vi "Speed_Ramp_test.vi"(3 "MaxRampRate":dbl, 4 "Input":dbl) -> (1 "Output":dbl)   [LabVIEW 2019]
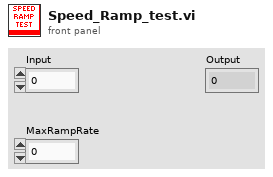
[diagram p1: front panel]
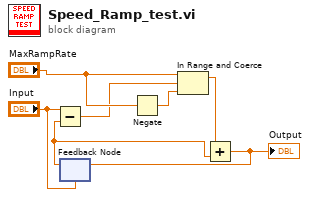
[diagram p0: block diagram]
diagram:
  n1 = feedback #1("Input") -> (w1:dbl)
  n2 = Subtract(x="Input", y=w1) -> (x-y=w5:dbl)
  n3 = Negate(x="MaxRampRate") -> (-x=w7:dbl)
  n4 = In Range and Coerce(upper limit="MaxRampRate", x=w5, lower limit=w7) -> (coerced(x)=w2:dbl)  [unwired: 1 out]
  n5 = Add(x=w2, y=w1) -> (x+y=w4:dbl)
  "Output" <- w4
  n6 = feedback-in #1(w4) -> ()
